vi "Write Direct Message Sent Msg.vi"(10 "Chat Window Model.lvlib:Direct Message Sent Msg.lvclass":refnum<class "Direct Message Sent Msg.lvclass">, 11 "Chat Window Model in":refnum<class "Chat Window Model.lvclass">) -> (3 "Chat Window Model out":refnum<class "Chat Window Model.lvclass">)   [LabVIEW 2014, in "Chat Window Model.lvlib" / "Chat Window Model.lvclass"]
uses:
  Chat Window Model.lvclass
  Chat Window Model Messages/Direct Message Sent Msg/Direct Message Sent Msg.lvclass
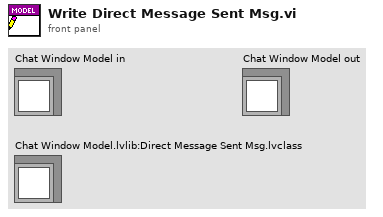
[diagram p1: front panel]
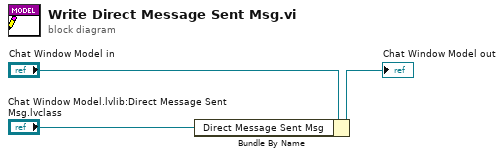
[diagram p0: block diagram]
diagram:
  n1 = Bundle By Name(cluster="Chat Window Model in", "Direct Message Sent Msg"="Chat Window Model.lvlib:Direct Message Sent Msg.lvclass") -> (→"Chat Window Model out":refnum<class "Chat Window Model.lvclass">)
